vi "Equations.vi"() -> ()   [LabVIEW 2020]
panel:
  out "y2":dbl
  out "y1":dbl
  in  "b":dbl
  in  "m":dbl
  in  "x":dbl
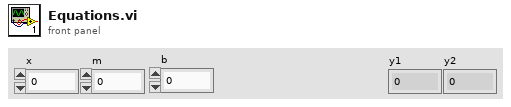
[diagram p1: front panel]
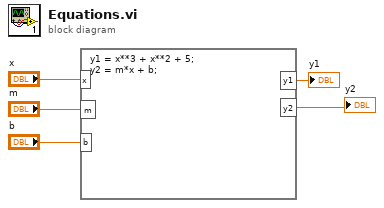
[diagram p0: block diagram]
diagram:
  n1 = formula code="y1 = x**3 + x**2 + 5;\ny2 = m*x + b;"("x"="x", "m"="m", "b"="b") -> ("y1"=→"y1":dbl, "y2"=→"y2":dbl)
